vi "AlliGator Check IRF.vi"(8 "Error In":errorcluster, 9 "SYNC Period":dbl[unit], 10 "Reference Decay":cluster{"t Array":dbl[], "IRF Array":dbl[]}, 11 "Current Decay":T1) -> (0 "Error Out":errorcluster, 2 "Reference Decay (or Dirac)":cluster{"t Array":dbl[], "IRF Array":dbl[]}, 3 "Current Decay (dup)":T1)   [LabVIEW 2021, in "AlliGator Decay Analysis.lvlib" / "AlliGator Decay Fit.lvlib"]
doc: "Check whether the provided IRF is a valid plot. If not, builds a mock Dirac IRF as a replacement."
uses:
  AlliGator Decay Fit.lvlib
  Arrays/Linear Ramp End Options.ctl
  14112560-ac03-4d9b-8c74-17f141675cd0.vi
  Graphs/XY Graph/XY Graph Add-Ons.lvlib
  Arrays/Arrays.lvlib
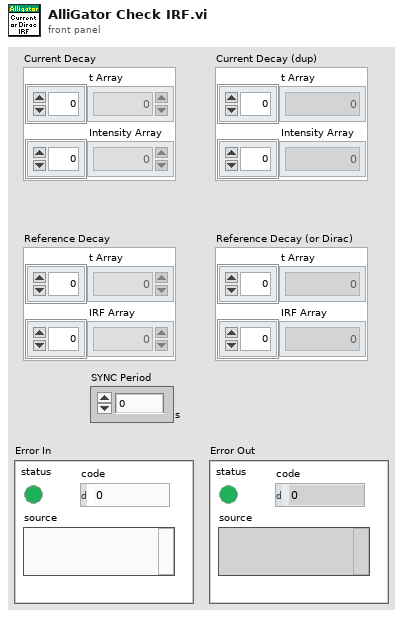
[diagram p1: front panel]
types:
  T1 = cluster{"t Array":dbl[], "Intensity Array":dbl[]}
  T2 = typedef "Arrays.lvlib/Linear Ramp End Options.ctl" = enum16{"Include Min/Exclude Max", "Exclude Min/Include Max", "Include Both Ends", "Exclude Both Ends"}
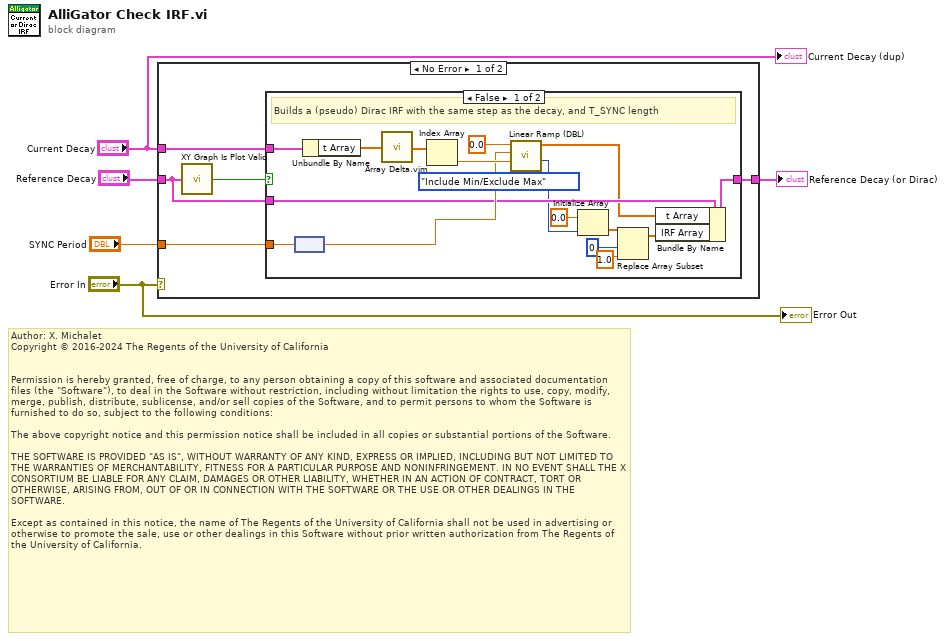
[diagram p0: block diagram]
diagram:
  # "Author: X. Michalet\nCopyright © 2016-2024 The Regents of the University of California\n \n\nPermission is hereby granted, free of charge, to any person obtaining a copy of this software and associated documentation files (the \"Software\"), to deal in the Software without restriction, including without limitation the rights to use, copy, modify, merge, publish, distribute, sublicense, and/or sell copies of the Software, and to permit persons to whom the Software is furnished to do so, subject to the following conditions:\n\nThe above copyright notice and this permission notice shall be included in all copies or substantial portions of the Software.\n\nTHE SOFTWARE IS PROVIDED \"AS IS\", WITHOUT WARRANTY OF ANY KIND, EXPRESS OR IMPLIED, INCLUDING BUT NOT LIMITED TO THE WARRANTIES OF MERCHANTABILITY, FITNESS FOR A PARTICULAR PURPOSE AND NONINFRINGEMENT. IN NO EVENT SHALL THE X CONSORTIUM BE LIABLE FOR ANY CLAIM, DAMAGES OR OTHER LIABILITY, WHETHER IN AN ACTION OF CONTRACT, TORT OR OTHERWISE, ARISING FROM, OUT OF OR IN CONNECTION WITH THE SOFTWARE OR THE USE OR OTHER DEALINGS IN THE SOFTWARE.\n\nExcept as contained in this notice, the name of The Regents of the University of California shall not be used in advertising or otherwise to promote the sale, use or other dealings in this Software without prior written authorization from The Regents of the University of California."
  n1 = case shown="No Error" "Error In" {
    tunnel: "Reference Decay" -> [w9 w29]
    tunnel: [w8 w29] -> w4
    tunnel: "SYNC Period" -> [w7 _]
    tunnel: "Current Decay" -> [w6 _]
    frame No Error {
      n2 = call "XY Graph Is Plot Valid.vi"("Plot"=w9) -> ("Is Valid Plot?"=w10:bool)  [unwired: 8 in]
      n3 = case shown="False" w10 {
        tunnel: w9 -> [w19 w28]
        tunnel: [w12 w28] -> w8
        tunnel: w7 -> [w25 _]
        tunnel: w6 -> [w27 _]
        frame False {
          # "Builds a (pseudo) Dirac IRF with the same step as the decay, and T_SYNC length"
          n4 = node(w25) -> (w20:dbl)
          n5 = Unbundle By Name(w27) -> ("t Array"=w26:dbl[])
          n6 = call "Array Delta.vim"("A"=w26) -> ("A[i+1]-A[i]"=w24:dbl[])  [unwired: 8 in]
          n7 = Index Array(array=w24) -> (element=w23:dbl)  [unwired: 1 in]
          n8 = call "Linear Ramp (DBL).vi"("Options"=Linear_Ramp_End_Options."Include Min/Exclude Max", "Delta"=w23, "Max"=w20, "Min"=0.0) -> ("# Elements"=w11:i32, "Ramp"=w18:dbl[])  [unwired: 6 in]
          n9 = Initialize Array(0.0 ("element"), w11) -> (w16:dbl[])
          n10 = Replace Array Subset(array=w16, new element=1.0 ("new element/subarray"), index=0) -> (w13:dbl[])
          n11 = Bundle By Name(cluster=w19, "t Array"=w18, "IRF Array"=w13) -> (w12:cluster{"t Array":dbl[], "IRF Array":dbl[]})
        }
        frame True {
        }
      }
    }
    frame Error {
    }
  }
  "Reference Decay (or Dirac)" <- w4
  "Current Decay (dup)" <- "Current Decay"
  "Error Out" <- "Error In"
